vi "Tx Channel Config Page.vi"(8 "error in (no error)":errorcluster, 11 "Node Ptr":T1 format="%.0x") -> (0 "error out":errorcluster)   [LabVIEW 2016, in "UDP-Custom-Device System Explorer.lvlib"]
uses:
  UDP-Custom-Device System Explorer.lvlib
  <vilib>/NI Veristand/Custom Device API/Custom Device Item Ref.ctl
  <vilib>/NI VeriStand/Custom Device API/Custom Device API.lvlib
  Property Accessors/Shared Channel Accessors.lvlib
  <vilib>/NI VeriStand/Custom Device Tools/Custom Device Utility Library/Custom Device Utility Library.lvlib
panel:
  out "Imported Channel Configuration":i32[](listbox) caption="Channels"
  in  "Channel Configuration File":path
  in  "Description":string
  out "Name":string
  in  "SHDocVw.IWebBrowser":refnum<k7>(container)
  in  "General Header":cluster{"Section Name":string}={"Section Name"="Channel Configuration"}
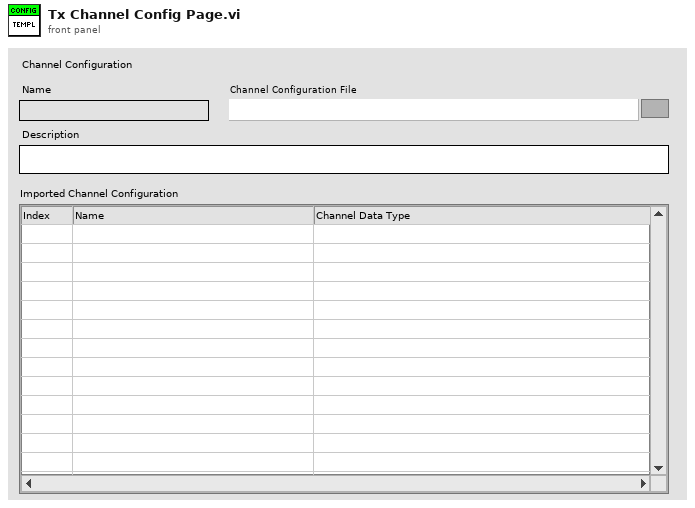
[diagram p1: front panel]
types:
  T1 = typedef "Custom Device API.lvlib/Custom Device Item Ref.ctl" = u64
  T2 = typedef "Custom Device API.lvlib/Custom Device Commands.ctl" = enum16{"Default", "Item renamed", "Shutdown", "Dynamic button pressed"}
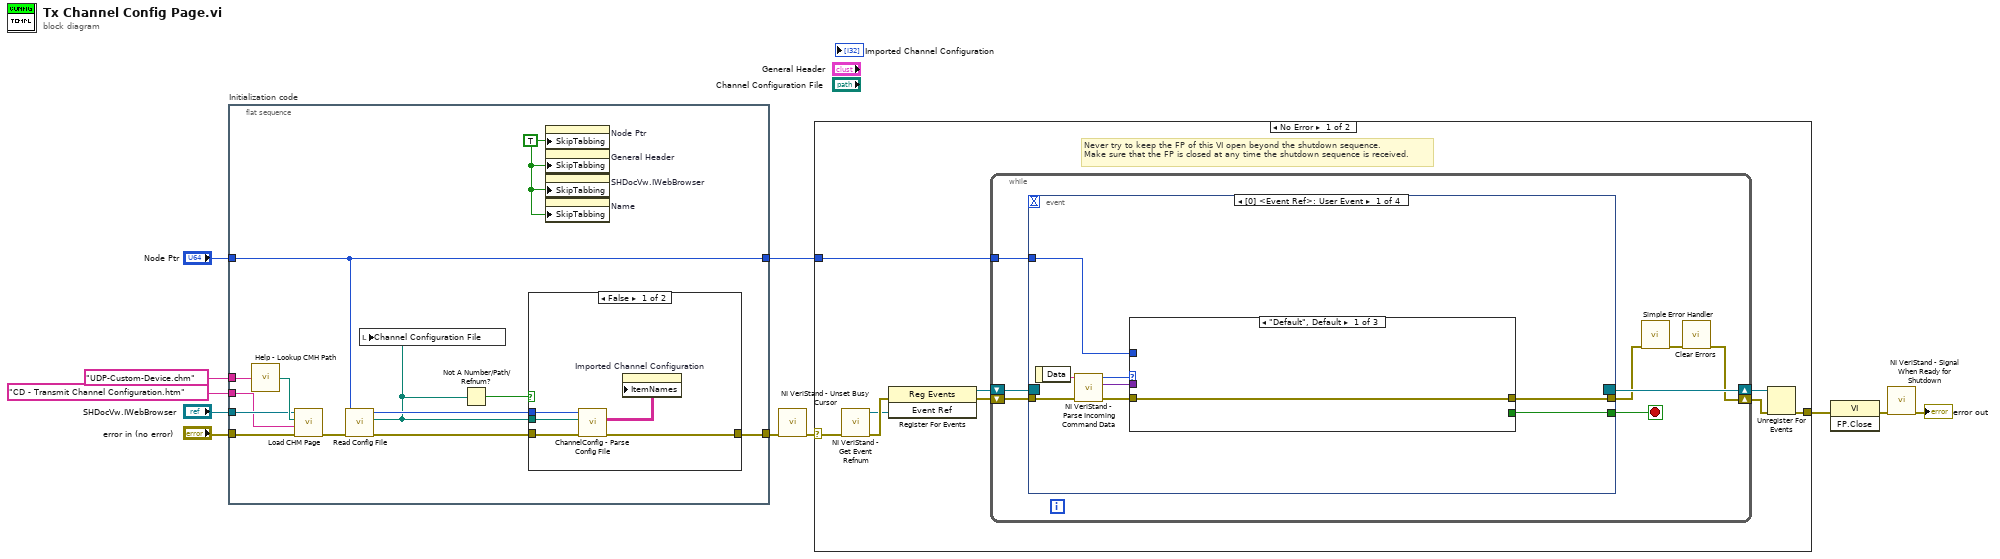
[diagram p0: block diagram]
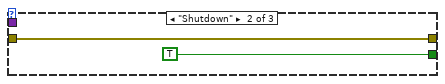
[diagram p3: hidden frame]
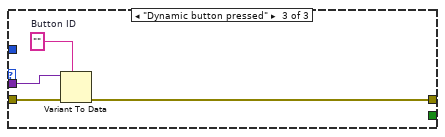
[diagram p4: hidden frame]
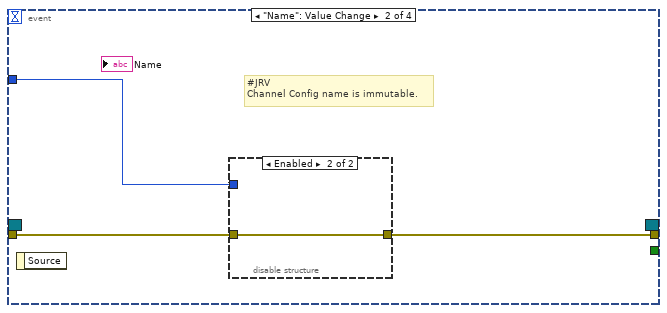
[diagram p5: hidden frame]
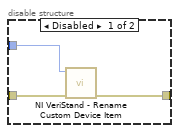
[diagram p6: hidden frame]
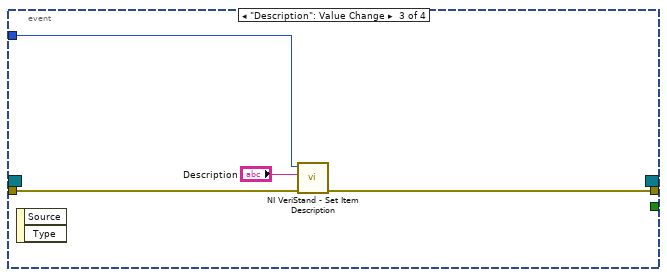
[diagram p7: hidden frame]
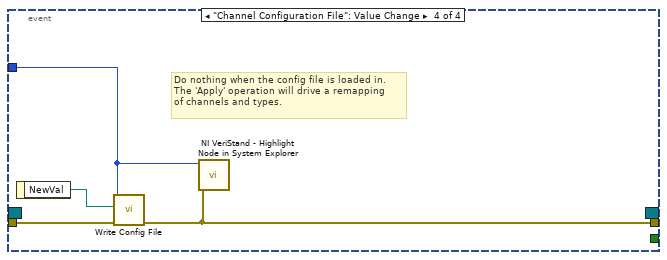
[diagram p8: hidden frame]
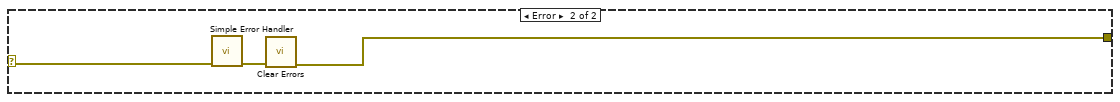
[diagram p9: hidden frame]
diagram:
  n1 = flat-sequence "Initialization code" {
    tunnel: "error in (no error)" -> [w23]
    tunnel: "Node Ptr" -> [w18]
    tunnel: [w13] -> w7
    tunnel: [w18] -> w4
    tunnel: "SHDocVw.IWebBrowser" -> [w22]
    tunnel: "CD - Transmit Channel Configuration.htm" ("CD_CHM_Section") -> [w20]
    tunnel: "UDP-Custom-Device.chm" ("CD_CHM_FileName") -> [w21]
    frame #0 {
      w12 = TRUE ("Skip When Tabbing")
      n2 = call "Help - Lookup CMH Path.vi"("Main CMH File"=w21) -> ("Compiled CMH Path"=w24:path)
      n3 = call <vilib>:"Load CHM Page.vi"("error in (no error)"=w23, "HTML File"=w20, "Compiled CHM Path"=w24, "Web Browser Reference"=w22) -> ("error out"=w19:errorcluster)  [unwired: 7 in]
      n4 = call "Read Config File.vi"("error in (no error)"=w19, "Node Ptr"=w18) -> ("error out"=w17:errorcluster, "Config File"=w14:path, "Node Ptr out"=w15:T1)  [unwired: 7 in]
      n5 = local write "Channel Configuration File"(w14) -> ()
      n6 = Not A Number/Path/Refnum?(number/path/refnum=w14) -> (NaN/Path/Refnum?=w16:bool)
      n7 = case shown="False" w16 {
        tunnel: w17 -> [w29 w30]
        tunnel: w15 -> [w28 _]
        tunnel: w14 -> [w27 _]
        tunnel: [w25 w30] -> w13
        frame False {
          n8 = call "ChannelConfig - Parse Config File.vi"("error in (no error)"=w29, "Config Path"=w27, "Node Ptr"=w28) -> ("error out"=w25:errorcluster, "Channel Configuration"=w26:string[][])  [unwired: 6 in, 1 out]
          n9 = property on="Imported Channel Configuration" class="MCListbox (strict)"("ItemNames"=w26) -> ()  [unwired: 2 in, 2 out]
        }
        frame True {
        }
      }
      n10 = property on="Node Ptr" class="DigNum (strict)"("SkipTabbing"=w12) -> ()  [unwired: 2 in, 2 out]
      n11 = property on="General Header" class="Clust (strict)"("SkipTabbing"=w12) -> ()  [unwired: 2 in, 2 out]
      n12 = property on="SHDocVw.IWebBrowser" class="AXCont"("SkipTabbing"=w12) -> ()  [unwired: 2 in, 2 out]
      n13 = property on="Name" class="Str"("SkipTabbing"=w12) -> ()  [unwired: 2 in, 2 out]
    }
  }
  n14 = call <vilib>:"NI VeriStand - Unset Busy Cursor.vi"("error in (no error)"=w7) -> ("error out"=w6:errorcluster)  [unwired: 10 out]
  n15 = case shown="No Error" w6 {
    selector: w6 -> [w31 w80]
    tunnel: [w36 w78] -> w11
    tunnel: w4 -> [w32 _]
    frame No Error {
      # "Never try to keep the FP of this VI open beyond the shutdown sequence.\nMake sure that the FP is closed at any time the shutdown sequence is received."
      n16 = call <vilib>:"NI VeriStand - Get Event Refnum.vi"("error in (no error)"=w31) -> ("error out"=w39:errorcluster, "Event Ref"=w35:refnum<user-event>)  [unwired: 9 out]
      n17 = register-events(error in=w39, w35) -> (reference out=w33:refnum<event-registration>, error out=w34:errorcluster)  [unwired: 1 in]
      n18 = while {
        tunnel: w32 -> [w43]
        shift-right: [w40] -> w37
        shift-left: w34 -> [w46]
        shift-right: [w47] -> w38
        shift-left: w33 -> [w45]
        stop <- w44 stop-if-true
        n19 = event shown="[0] <Event Ref>: User Event" {
          selector: w45 -> [_ _ _ _]
          dyn-events: [_ _ _ _] -> w47
          timeout: _ -> [_ _ _ _]
          tunnel: w46 -> [w55 w65 w73 w75]
          tunnel: [w51 _ _ _] -> w44
          tunnel: [w50 w63 w70 w74] -> w42
          tunnel: w43 -> [w49 w64 w72 w77]
          event User Event {
            n20 = event-data() -> ("Data"=w54:string)  [unwired: 1 out]
            n21 = call <vilib>:"NI VeriStand - Parse Incoming Command Data.vi"("error in (no error)"=w55, "Incoming data"=w54) -> ("error out"=w53:errorcluster, "Outgoing data"=w48:variant, "Action"=w52:T2)  [unwired: 7 out]
            n22 = case shown="\"Default\", Default" w52 {
              tunnel: w53 -> [w56 w57 w62]
              tunnel: [_ TRUE _] -> w51
              tunnel: [w56 w57 w59] -> w50
              tunnel: w49 -> [_ _ _]
              tunnel: w48 -> [_ _ w61]
              frame "Default", Default {
              }
              frame "Shutdown" {
              }
              frame "Dynamic button pressed" {
                w60 = ""  # Button ID
                n23 = Variant To Data(error in=w62, type=w60, Variant=w61) -> (error out=w59:errorcluster)  [unwired: 1 out]
              }
            }
          }
          event "Name": Value Change {
            # "#JRV\nChannel Config name is immutable."
            n24 = event-data() -> ()  [unwired: 2 out]
            n25 = disable-structure shown="Enabled" {
              disable-tunnel: w65 -> [w68 w69]
              disable-tunnel: w64 -> [w67 _]
              disable-tunnel: [w66 w69] -> w63
              frame Disabled {
                n26 = call <vilib>:"NI VeriStand - Rename Custom Device Item.vi"("error in (no error)"=w68, "Item Ref in"=w67) -> ("error out"=w66:errorcluster)  [unwired: 7 in, 2 out]
              }
              frame Enabled {
              }
            }
          }
          event "Description": Value Change {
            n27 = event-data() -> ()  [unwired: 3 out]
            n28 = call <vilib>:"NI VeriStand - Set Item Description.vi"("error in (no error)"=w73, "Description"="Description", "Item Ref in"=w72) -> ("error out"=w70:errorcluster)  [unwired: 6 in, 2 out]
          }
          event "Channel Configuration File": Value Change {
            # "Do nothing when the config file is loaded in.\nThe 'Apply' operation will drive a remapping\nof channels and types."
            n29 = event-data() -> ("NewVal"=w76:path)  [unwired: 1 out]
            n30 = call "Write Config File.vi"("error in (no error)"=w75, "Config File"=w76, "Node Ptr"=w77) -> ("error out"=w74:errorcluster)  [unwired: 7 in, 1 out]
            n31 = call <vilib>:"NI VeriStand - Highlight Node in System Explorer.vi"("error in (no error)"=w74, "Item Ref in"=w77) -> ()  [unwired: 8 in, 2 out]
          }
        }
        n32 = call <vilib>:"Simple Error Handler.vi"("error in (no error)"=w42) -> ("error out"=w41:errorcluster)  [unwired: 1 in, 7 out]
        n33 = call <vilib>:"Clear Errors.vi"("error in (no error)"=w41) -> ("error out"=w40:errorcluster)  [unwired: 1 in, 5 out]
      }
      n34 = Unregister For Events(event registration refnum=w38, error in=w37) -> (error out=w36:errorcluster)
    }
    frame Error {
      n35 = call <vilib>:"Simple Error Handler.vi"("error in (no error)"=w80) -> ("error out"=w79:errorcluster)  [unwired: 1 in, 7 out]
      n36 = call <vilib>:"Clear Errors.vi"("error in (no error)"=w79) -> ("error out"=w78:errorcluster)  [unwired: 1 in, 5 out]
    }
  }
  n37 = invoke class="VI" method="FP.Close"(error in=w11) -> (error out=w10:errorcluster)  [unwired: 2 in, 2 out]
  n38 = call <vilib>:"NI VeriStand - Signal When Ready for Shutdown.vi"("error in (no error)"=w10) -> ("error out"=→"error out":errorcluster)  [unwired: 10 out]
